vi "Push Error if Different.vi"(1 "error in":errorcluster, 2 "Error Q":refnum<queue>) -> ()   [LabVIEW 2016, in "Ballard Arinc-429 Engine.lvlib"]
uses:
  Ballard Arinc-429 Engine.lvlib
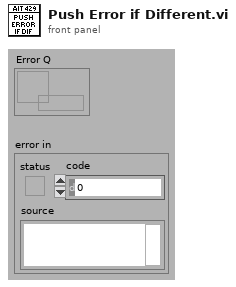
[diagram p1: front panel]
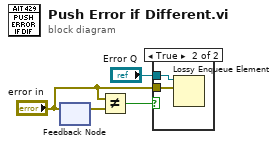
[diagram p0: block diagram]
diagram:
  n1 = feedback #1() -> (w1:errorcluster)  [unwired: 1 in]
  n2 = feedback-in #1("error in") -> ()
  n3 = Not Equal?(x="error in", y=w1) -> (x != y?=w3:bool)
  n4 = case shown="True" w3 {
    tunnel: "error in" -> [_ w6]
    tunnel: "Error Q" -> [_ w5]
    frame False {
    }
    frame True {
      n5 = Lossy Enqueue Element(queue=w5, element=w6) -> ()  [unwired: 1 in, 4 out]
    }
  }
